vi "Build Address Frame.vi"(0 "RFFE Extended Command in":refnum<class "RFFE Extended Command.lvclass">, 11 "error in (no error)":errorcluster) -> (4 "RFFE Extended Command out":refnum<class "RFFE Extended Command.lvclass">, 6 "Address Frame":u8[](array[numeric]), 15 "error out":errorcluster)   [LabVIEW 2018, in "MIPI RFFE API.lvlib" / "RFFE Extended Command.lvclass"]
uses:
  RFFE Extended Command.lvclass
  C:/Users/semoore/Projects/mipi-rffe-labview-oop/Command/RFFE Command.lvclass
  Command/RFFE Command.lvclass/RFFE Command.ctl
  Command/Get Register Address.vi
  MIPI RFFE API.lvlib
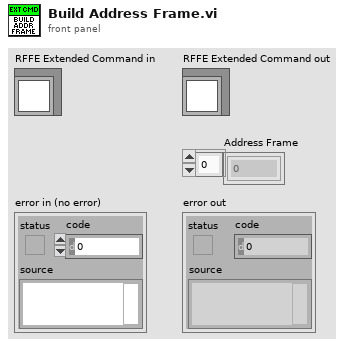
[diagram p1: front panel]
types:
  T1 = typedef "RFFE Commands.lvlib/Register Address.ctl" = u16
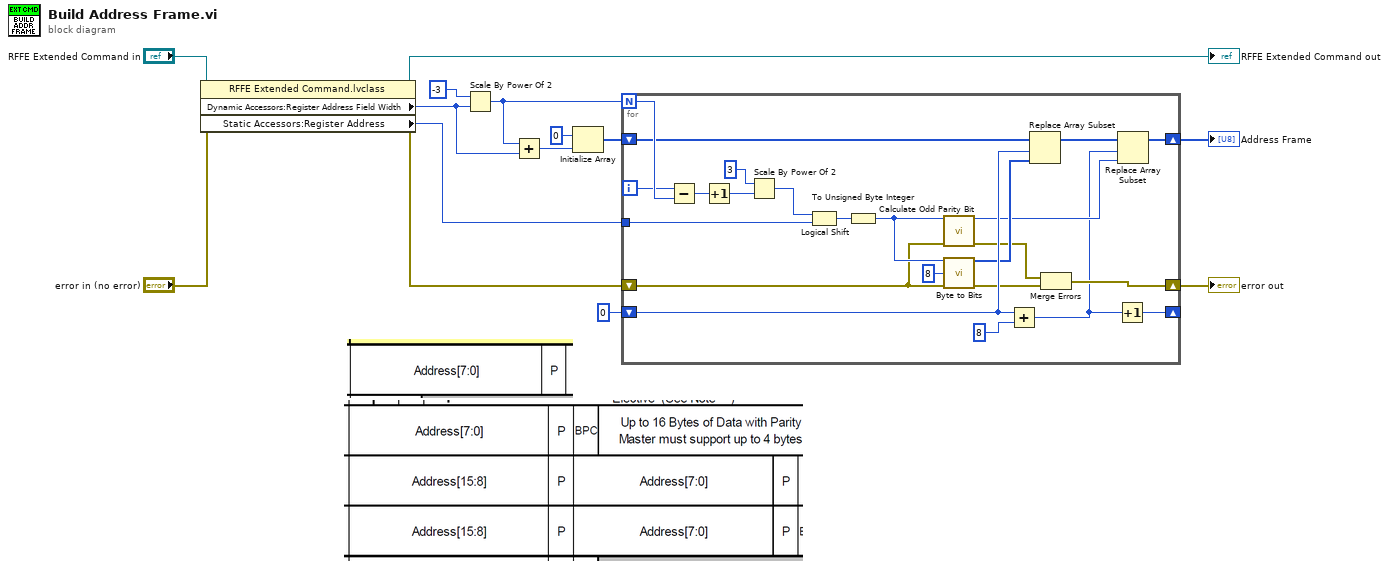
[diagram p0: block diagram]
diagram:
  n1 = property class="RFFE Extended Command.lvclass"(reference="RFFE Extended Command in", error in="error in (no error)") -> (reference out=→"RFFE Extended Command out":refnum<class "RFFE Extended Command.lvclass">, error out=w6:errorcluster, "Dynamic Accessors:Register Address Field Width"=w2:i32, "Static Accessors:Register Address"=w4:T1)
  n2 = Scale By Power Of 2(n=i16 -3, x=w2) -> (x*2^n=w1:i32)
  n3 = Add(x=w1, y=w2) -> (x+y=w5:i32)
  n4 = Initialize Array(u8 0 ("unsigned 8bit integer"), w5) -> (w7:u8[])
  n5 = for {
    N: w1 -> [w35]
    shift-right: [w15] -> _
    shift-left: 0 ("y") -> [w27]
    tunnel: w4 -> [w37]
    shift-right: [w18] -> w10
    shift-left: w7 -> [w28]
    shift-right: [w20] -> w12
    shift-left: w6 -> [w23]
    i -> [w34]
    n6 = Subtract(x=w34, y=w35) -> (x-y=w33:i32)
    n7 = Increment(x=w33) -> (x+1=w32:i32)
    n8 = Scale By Power Of 2(n=i16 3, x=w32) -> (x*2^n=w30:i32)
    n9 = Logical Shift(y=w30, x=w37) -> (x << y=w36:T1)
    n10 = To Unsigned Byte Integer(number=w36) -> (unsigned 8bit integer=w24:u8)
    n11 = call "Calculate Odd Parity Bit.vi"("Byte"=w24, "error in (no error)"=w23) -> ("Odd Parity Bit"=w17:u8, "error out"=w21:errorcluster)  [unwired: 12 in]
    n12 = call "Byte to Bits.vi"("Byte"=w24, "Bit Width"=8, "error in (no error)"=w23) -> ("Bits"=w26:u8[], "error out"=w22:errorcluster)  [unwired: 11 in]
    n13 = Add(x=w27, y=8) -> (x+y=w16:i32)
    n14 = Replace Array Subset(array=w28, new element=w26, index=w27) -> (w19:u8[])
    n15 = Merge Errors(w21, w22) -> (w20:errorcluster)
    n16 = Increment(x=w16) -> (x+1=w15:i32)
    n17 = Replace Array Subset(array=w19, new element=w17, index=w16) -> (w18:u8[])
  }
  "error out" <- w12
  "Address Frame" <- w10
